vi "theta_to_torque.vi"(8 "error in (no error)":errorcluster, 11 "Motor angle (deg)":dbl) -> (0 "error out":errorcluster, 3 "Torque fraction [-1:1]":dbl)   [LabVIEW 2018]
doc: "This VI converts theta angle to the respective torque angle for the Winchester type motor."
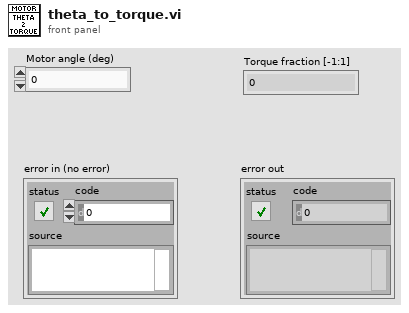
[diagram p1: front panel]
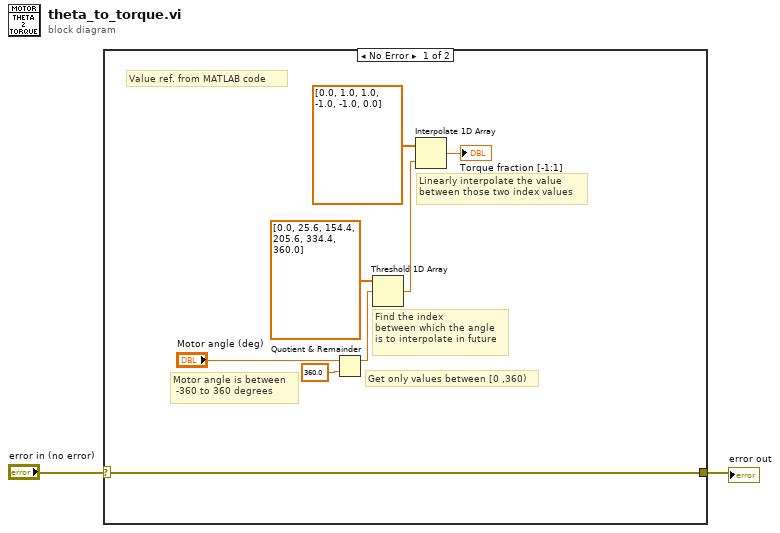
[diagram p0: block diagram]
diagram:
  n1 = case shown="No Error" "error in (no error)" {
    selector: "error in (no error)" -> [w4 w11]
    tunnel: [w4 w11] -> w1
    frame No Error {
      # "Motor angle is between\n -360 to 360 degrees"
      # "Value ref. from MATLAB code"
      # "Linearly interpolate the value\nbetween those two index values"
      # "Find the index \nbetween which the angle\nis to interpolate in future"
      # "Get only values between [0 ,360)"
      n2 = Quotient & Remainder(x="Motor angle (deg)", y=360.0) -> (x-y*floor(x/y)=w10:dbl)  [unwired: 1 out]
      n3 = Threshold 1D Array(2:w10, 3:dbl[] [0.0, 25.6, 154.4, 205.6, 334.4, 360.0] ("array of numbers or points")) -> (0:w9:dbl)  [unwired: 1 in]
      n4 = Interpolate 1D Array(1:w9, 2:dbl[] [0.0, 1.0, 1.0, -1.0, -1.0, 0.0] ("array of numbers or points")) -> (0:→"Torque fraction [-1:1]":dbl)
    }
    frame Error {
    }
  }
  "error out" <- w1
